vi "FPGA Main_v2.vi"() -> ()   [LabVIEW 2019]
doc: "Main FPGA VI\nUse the bitfile generated by this VI in the real-time code.\n\nFlip the channels for input and output"
uses:
  TypeDefs/SamplingModeEnum.ctl
  TypeDefs/AO mode TabCtrl.ctl
  <vilib>/rvi/Emulation/niFpgaGetClockAttributes.vi
  <vilib>/rvi/Emulation/niFpgaSctlEmulationGetInTimedLoop.vi
  <vilib>/rvi/Emulation/niFpgaEmulationReportErrorSimple.vi
  <vilib>/rvi/eio/common/nirviEmuTemplateMethod_errors.vi
  <vilib>/rvi/Emulation/niFpgaEmulationIsFPGAContextNoSignature.vi
  <vilib>/rvi/errors/niFpgaSetErrorForExecOnDevCompSimple.vi
  <vilib>/rvi/eio/common/nirviEmuReportErrorAndStop.vi
  <vilib>/rvi/DataTransferAndStorage/Container/Common/niFpgaContainerGetUniqueNameForEmu.vi
  <vilib>/rvi/FIFO/Fifo_Resource/nirvififoEmulationSetSize.vi
  <vilib>/rvi/FIFO/Fifo_Resource/nirviFifoEmulationQueueMgr.vi
  <instcachedir>/0/nirviFifoEmulationQueueMgr_E5CAEC123FF24DC58D834DCA3CDAA9B5.lvgen/nirviFifoEmulationQueueMgr_E5CAEC123FF24DC58D834DCA3CDAA9B5_003.vi
  <vilib>/rvi/FIFO/Fifo_Resource/nirvififoEmulationDetermineInputValidOut.vi
  <vilib>/rvi/FIFO/Fifo_Resource/nirvififoEmulationCreateLock.vi
  <vilib>/rvi/Emulation/niFpgaProcessEmulError.vi
  <vilib>/rvi/FIFO/Fifo_Resource/nirvififoEmulationObtainLock.vi
  <vilib>/rvi/FIFO/Fifo_Resource/nirvififoEmulationReleaseLock.vi
  <vilib>/rvi/occurrence/nirviWaitOnOccurrenceBase.vi
  <vilib>/rvi/errors/nirviReportUnexpectedCaseInternalError.vi
  <vilib>/rvi/errors/nirviReportUnexpectedCaseInternalError (U32).vi
  <vilib>/rvi/Emulation/niFpgaCriticalErrorInLSC.vi
  <vilib>/Utility/error.llb/Clear Errors.vi
  <vilib>/eio/EIONode/EIONode.xnode
  <vilib>/rvi/Analysis/measure/butterworth/XNode/niFpgaButterworthFilter.xnode
  <vilib>/rvi/FXPMathLib/FxpMul/XNode/nifxpmath_Multiplier.xnode
  <vilib>/rvi/DataTransferAndStorage/Container/XNode/niFpgaContainer.xnode
  <vilib>/rvi/FIFO/Fifo_Resource/nirvififoEmulationWrite.vi
  <vilib>/rvi/FIFO/Fifo_Resource/nirvififoEmulationRead.vi
  FPGA functions/FPGA functions.lvlib
  <vilib>/rvi/FXPMathLib/sim/FxpSim.dll
panel:
  in  "AO mode":T1
  in  "AO Out [V]":fxp<+/-,18,5> format="%#.6g"
  in  "Scaled Butterworth Coeffs":i32[](array[numeric])=[-1036986264, 2110353124, 93741, -1058362983, 2131726043, 94691]
  in  "Sampling Mode":T2
  out "Int. Output":i16
  out "Raw Int. Input":i16
  in  "Bit-resolution":i8=12
  in  "Sample Time [ticks]":u32=120
  out "AO Loop time [ticks]":u32
  in  "AO enable?":bool
  out "AI In [V]":fxp<+/-,25,5> format="%#.6g"
  out "AI Loop time [ticks]":u32
  out "FPGA AO DMA\nOverflow?":bool
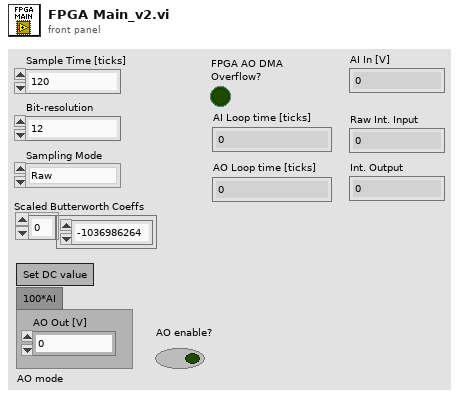
[diagram p1: front panel]
types:
  T1 = typedef "AO mode TabCtrl.ctl" = enum32{"Set DC value", "100*AI"}
  T2 = typedef "SamplingModeEnum.ctl" = enum16{"Raw", "LPF", "4 pt. Avg. + LPF"}
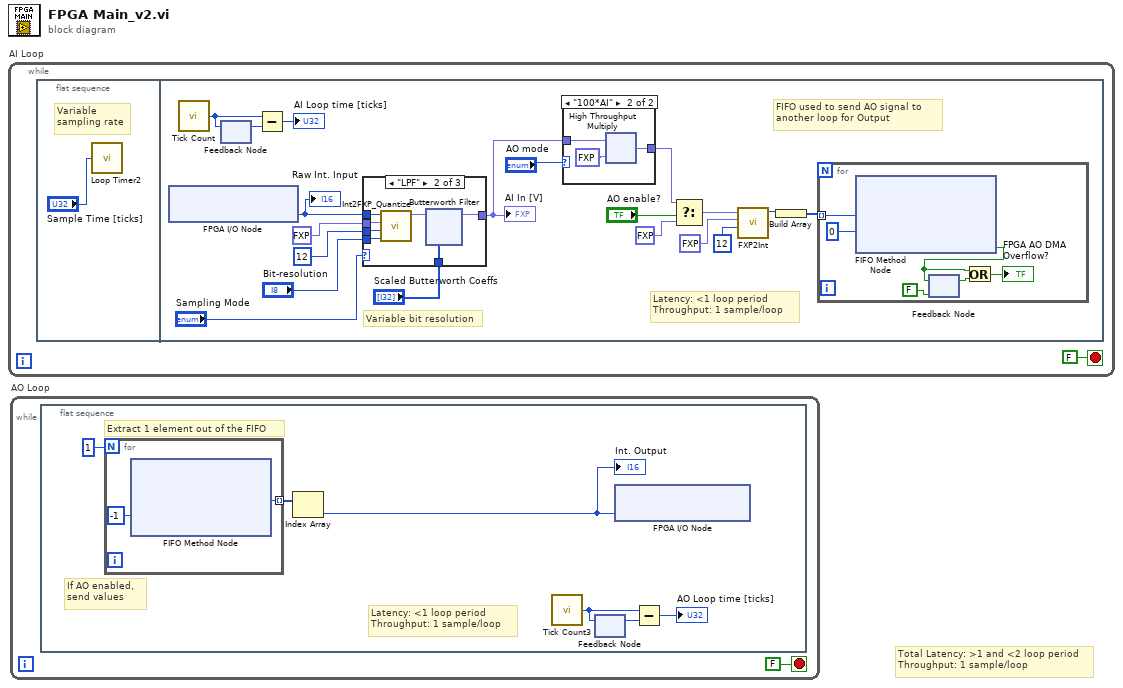
[diagram p0: block diagram]
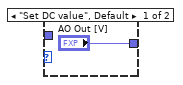
[diagram p2: hidden frame]
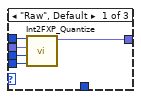
[diagram p3: hidden frame]
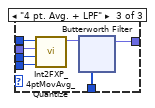
[diagram p4: hidden frame]
diagram:
  # "Total Latency: >1 and <2 loop period\nThroughput: 1 sample/loop"
  n1 = while "AI Loop" {
    stop <- FALSE stop-if-true
    n2 = flat-sequence {
      frame #0 {
        # "Variable\nsampling rate"
        n3 = call "Loop Timer2"("Count(Ticks)"="Sample Time [ticks]") -> ()  [unwired: 1 out]
      }
      frame #1 {
        # "Variable bit resolution"
        # "Latency: <1 loop period\nThroughput: 1 sample/loop"
        # "FIFO used to send AO signal to \nanother loop for Output"
        n4 = xnode "FPGA I/O Node"() -> ("ConnectorC/AI0"=w7:i16)  [unwired: 1 in, 1 out]
        "Raw Int. Input" <- w7
        n5 = call "Tick Count"() -> ("Tick Count(Ticks)"=w21:u32)
        n6 = feedback #1() -> (w20:u32)  [unwired: 1 in]
        n7 = feedback-in #1(w21) -> ()
        n8 = Subtract(x=w21, y=w20) -> (x-y=→"AI Loop time [ticks]":u32)
        n9 = case shown="\"LPF\"" "Sampling Mode" {
          tunnel: [w30 w35 w48] -> w4
          tunnel: i8 12 ("Input Bit resolution") -> [w29 w32 w51]
          tunnel: fxp<+,8,4> 10.0 ("Multiplier") -> [w28 w33 w52]
          tunnel: "Bit-resolution" -> [w27 w31 w50]
          tunnel: w7 -> [w26 w37 w47]
          tunnel: "Scaled Butterworth Coeffs" -> [_ w34 w46]
          frame "Raw", Default {
            n10 = call "Int2FXP_Quantize.vi"("Output Bit resolution"=w27, "Input Bit resolution"=w29, "Multiplier"=w28, "Input (Int)"=w26) -> ("Output (FXP)"=w30:fxp<+/-,25,5>)  [unwired: 7 in]
          }
          frame "LPF" {
            n11 = call "Int2FXP_Quantize.vi"("Output Bit resolution"=w31, "Input Bit resolution"=w32, "Multiplier"=w33, "Input (Int)"=w37) -> ("Output (FXP)"=w36:fxp<+/-,25,5>)  [unwired: 7 in]
            n12 = xnode "Butterworth Filter"("input data"=w36, "scaled coefficients"=w34) -> ("output data"=w35:fxp<+/-,25,5>)  [unwired: 1 in]
          }
          frame "4 pt. Avg. + LPF" {
            n13 = call "Int2FXP_4ptMovAvg_Quantize.vi"("Output Bit resolution"=w50, "Input Bit resolution"=w51, "Multiplier"=w52, "Input (Int)"=w47) -> ("Output (FXP)"=w49:fxp<+/-,25,5>)  [unwired: 7 in]
            n14 = xnode "Butterworth Filter"("input data"=w49, "scaled coefficients"=w46) -> ("output data"=w48:fxp<+/-,25,5>)  [unwired: 1 in]
          }
        }
        "AI In [V]" <- w4
        n15 = case shown="\"100*AI\"" "AO mode" {
          tunnel: ["AO Out [V]" w23] -> w8
          tunnel: w4 -> [_ w25]
          frame "Set DC value", Default {
          }
          frame "100*AI" {
            n16 = xnode ("High Throughput Multiply")("x"=w25, "y"=fxp<+,5,7> 100.0) -> ("x*y"=w23:fxp<+/-,18,5>)
          }
        }
        n17 = Select(t=w8, s="AO enable?", f=fxp<+/-,18,5> 0.0) -> (s? t:f=w9:fxp<+/-,18,5>)
        n18 = call "FXP2Int.vi"("Output Bit resolution"=i8 12 ("Bit resolution"), "Multiplier"=fxp<+,18,-1> 0.10000038146972656, "Input (FXP)"=w9) -> ("Output (Int)"=w18:i16)  [unwired: 8 in]
        n19 = Build Array(w18) -> (w11:i16[])
        n20 = for {
          tunnel: w11 -> [w63] mode=indexing
          n21 = xnode ("FIFO Method Node")("Element"=w63, "Timeout"=0) -> ("Timed Out?"=w61:bool)  [unwired: 1 in, 1 out]
          n22 = feedback-in #2(w61) -> ()
          n23 = feedback #2(FALSE ("Timed Out?")) -> (w65:bool)
          n24 = Or(x=w61, y=w65) -> (x .or. y?=→"FPGA AO DMA\nOverflow?":bool)
        }
      }
    }
  }
  n25 = while "AO Loop" {
    stop <- FALSE stop-if-true
    n26 = flat-sequence {
      frame #0 {
        # "Latency: <1 loop period\nThroughput: 1 sample/loop"
        # "If AO enabled, \nsend values"
        # "Extract 1 element out of the FIFO"
        n27 = for {
          N: 1 -> [_]
          tunnel: [w75] -> w70 mode=indexing
          n28 = xnode ("FIFO Method Node")("Timeout"=-1) -> ("Element"=w75:i16)  [unwired: 1 in, 2 out]
        }
        n29 = Index Array(array=w70) -> (element=w68:i16)  [unwired: 1 in]
        "Int. Output" <- w68
        n30 = call "Tick Count3"() -> ("Tick Count(Ticks)"=w73:u32)
        n31 = feedback #3() -> (w72:u32)  [unwired: 1 in]
        n32 = feedback-in #3(w73) -> ()
        n33 = xnode "FPGA I/O Node"("ConnectorC/AO0"=w68) -> ()  [unwired: 1 in, 1 out]
        n34 = Subtract(x=w73, y=w72) -> (x-y=→"AO Loop time [ticks]":u32)
      }
    }
  }
